vi "L1_RegisterDump_File_Appender.vi"(0 "file path (dialog if empty)":path, 1 "Dec Value":i32, 2 "Register Default":i32, 3 "Register Number":i32) -> ()   [LabVIEW 2012]
uses:
  <vilib>/Utility/file.llb/Write To Spreadsheet File (string).vi
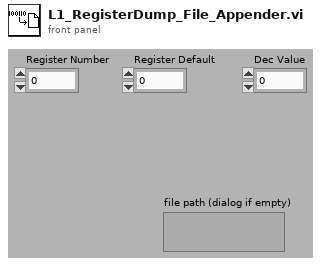
[diagram p1: front panel]
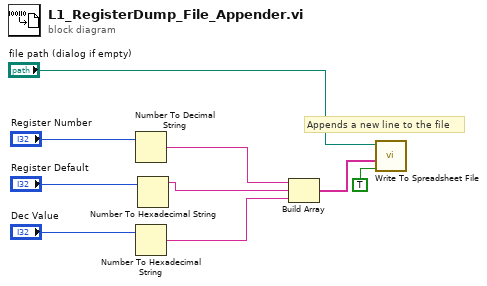
[diagram p0: block diagram]
diagram:
  # "Appends a new line to the file"
  n1 = Number To Decimal String(number="Register Number") -> (decimal integer string=w6:string)  [unwired: 1 in]
  n2 = Number To Hexadecimal String(2:"Dec Value") -> (0:w2:string)  [unwired: 1 in]
  n3 = Number To Hexadecimal String(2:"Register Default") -> (0:w1:string)  [unwired: 1 in]
  n4 = Build Array(w6, w1, w2) -> (w8:string[])
  n5 = call-poly <vilib>:"Write To Spreadsheet File.vi"("append to file? (new file:F)"=TRUE, "1D data"=w8, "file path (dialog if empty)"="file path (dialog if empty)") -> ()  [unwired: 5 in, 1 out]
